vi "ChannelEncode.vi"(8 "error in (no error)":errorcluster, 10 "Code Cluster":T1={"Code type"=enum."No code", "Encode factor"=2, "Constraint length(For convolution code)"=3}, 11 "Uncode bits":i8[](array[numeric])) -> (0 "error out":errorcluster, 3 "Encoded bits":i8[](array[numeric]))   [LabVIEW 2013]
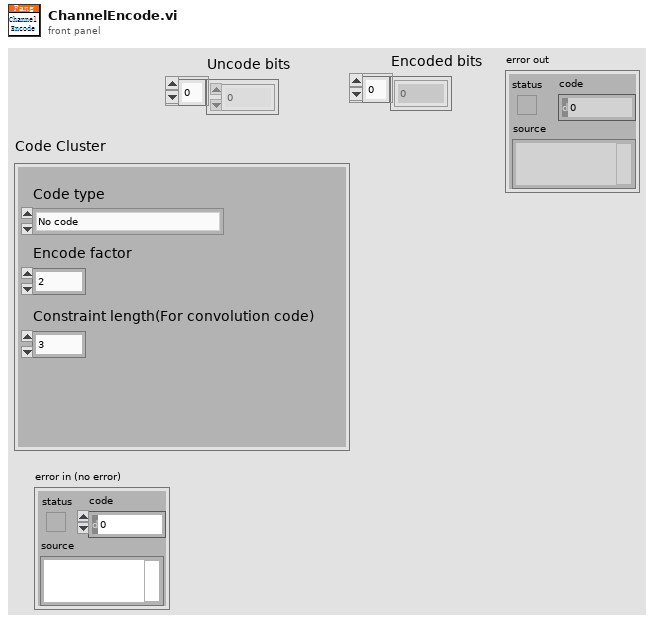
[diagram p1: front panel]
types:
  T1 = cluster{"Code type":enum16{"No code", "Convolution code", "Repetition code"}, "Encode factor":i32, "Constraint length(For convolution code)":i32}
  T2 = enum16{"No code", "Convolution code", "Repetition code"}
  T3 = cluster{"constraint length (K)":i32, "initial state":u32, "Encode factor":i32}
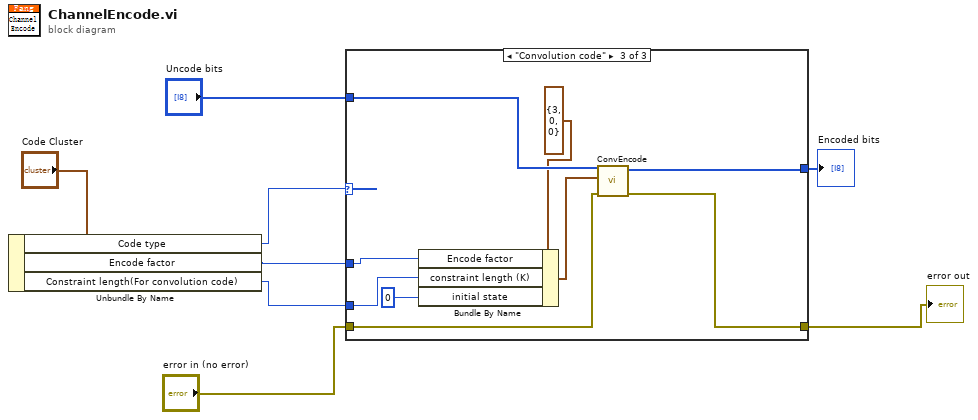
[diagram p0: block diagram]
diagram:
  n1 = Unbundle By Name("Code Cluster") -> ("Code type"=w5:T2, "Encode factor"=w4:i32, "Constraint length(For convolution code)"=w3:i32)
  n2 = case shown="\"Convolution code\"" w5 {
    tunnel: "Uncode bits" -> [w10 w14 w27]
    tunnel: w4 -> [_ w13 w20]
    tunnel: [w10 w12 w23] -> w7
    tunnel: w3 -> [_ _ w22]
    tunnel: "error in (no error)" -> [w9 w11 w25]
    tunnel: [w9 w11 w24] -> w1
    frame "No code", Default {
    }
    frame "Repetition code" {
      n3 = for {
        tunnel: w14 -> [w16] mode=indexing
        tunnel: w13 -> [w17]
        tunnel: [w15] -> w12 mode=concatenating
        n4 = for {
          N: w17 -> [_]
          tunnel: w16 -> [w18]
          tunnel: [w18] -> w15 mode=indexing
        }
      }
    }
    frame "Convolution code" {
      n5 = Bundle By Name(cluster=T3 {"constraint length (K)"=3, "initial state"=0, "Encode factor"=0} ("Encode Parameter"), "Encode factor"=w20, "constraint length (K)"=w22, "initial state"=u32 0) -> (w19:T3)
      n6 = call "ConvEncode.vi"("error in (no error)"=w25, "Encode Parameter"=w19, "Input Bits"=w27) -> ("error out"=w24:errorcluster, "output bit stream"=w23:i8[])  [unwired: 7 in]
    }
  }
  "Encoded bits" <- w7
  "error out" <- w1
